vi "MoveLogic.vi"() -> ()   [LabVIEW 2016]
uses:
  Control 1.ctl
panel:
  in  "Array 3":i32[](array[numeric])
  in  "Array":T1
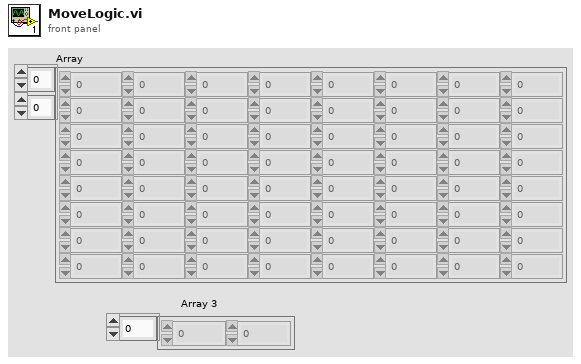
[diagram p1: front panel]
types:
  T1 = typedef "Control 1.ctl" = i32[][]
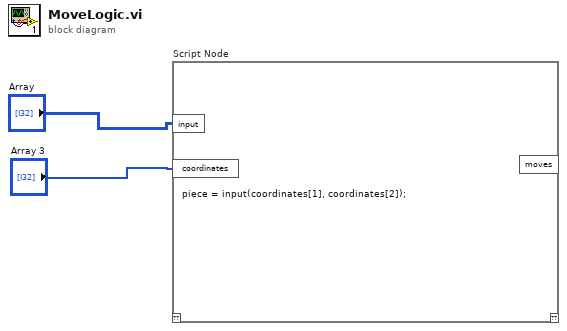
[diagram p0: block diagram]
diagram:
  n1 = script code="piece = input(coordinates[1], coordinates[2]);" "Script Node"("input"="Array", "coordinates"="Array 3") -> ()  [unwired: 1 in, 2 out]
